vi "Reconnect.vi"(8 "error in (no error)":errorcluster, 11 "TCP Stream in":refnum<class "TCP Stream.lvclass">) -> (0 "error out":errorcluster, 3 "TCP Stream out":refnum<class "TCP Stream.lvclass">)   [LabVIEW 2020, in "Stream-TCP.lvlib" / "TCP Stream.lvclass"]
uses:
  TCP Stream.lvclass
  TCP Stream.lvclass/TCP Stream.ctl
  Client Command.ctl
  Stream-TCP.lvlib
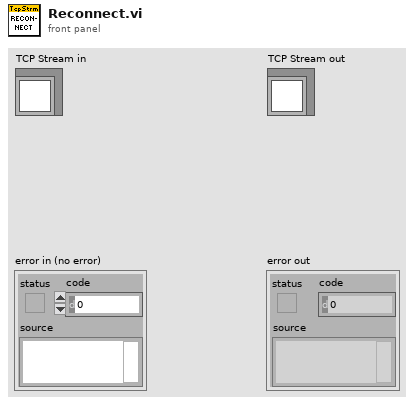
[diagram p1: front panel]
types:
  T1 = typedef "Stream-TCP.lvlib/Client Command.ctl" = enum16{"Connect", "Close", "Shutdown", "Reconnect"}
  T2 = typedef "Stream-TCP.lvlib/TCP Stream.lvclass/Ref Data.ctl" = cluster{"Client Command Queue":T3}
  T3 = typedef "Stream-TCP.lvlib/Client Command Queue.ctl" = refnum<queue>
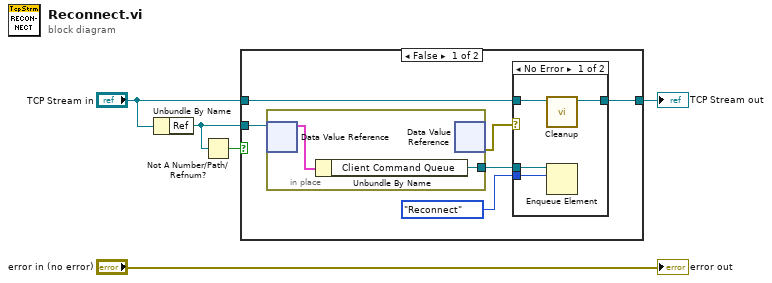
[diagram p0: block diagram]
diagram:
  n1 = Unbundle By Name("TCP Stream in") -> ("Ref"=w2:refnum<data-value>)
  n2 = Not A Number/Path/Refnum?(number/path/refnum=w2) -> (NaN/Path/Refnum?=w1:bool)
  n3 = case shown="False" w1 {
    tunnel: "TCP Stream in" -> [w9 w19]
    tunnel: [w8 w19] -> w3
    tunnel: w2 -> [w6 _]
    frame False {
      n4 = in-place {
        in-place-border: [w17] -> w11
        n5 = in-place-dvr #1(w6) -> (w18:T2)  [unwired: 1 out]
        n6 = Unbundle By Name(w18) -> ("Client Command Queue"=w17:T3)
        n7 = in-place-dvr #1() -> (w7:errorcluster)  [unwired: 1 in, 1 out]
      }
      n8 = case shown="No Error" w7 {
        tunnel: w11 -> [w15 _]
        tunnel: Client_Command."Reconnect" ("element") -> [w14 _]
        tunnel: w9 -> [w13 w16]
        tunnel: [w12 w16] -> w8
        frame No Error {
          n9 = call "Cleanup.vi"("TCP Stream in"=w13) -> ("TCP Stream out"=w12:refnum<class "TCP Stream.lvclass">)  [unwired: 9 in, 1 out]
          n10 = Enqueue Element(queue=w15, element=w14) -> ()  [unwired: 2 in, 3 out]
        }
        frame Error {
        }
      }
    }
    frame True {
    }
  }
  "TCP Stream out" <- w3
  "error out" <- "error in (no error)"
